vi "RSZVB Query Extension Unit Hardware Options.vi"(8 "error in (no error)":errorcluster {"code" format="%.0x"}, 11 "VISA session":refnum<visa-resource-name>) -> (0 "error out":errorcluster {"code" format="%.0x"}, 1 "Options":string, 3 "dup VISA session":refnum<visa-resource-name>)   [LabVIEW 2011]
doc: "Queries the hardware options of a connected extension unit ZVAXxx.\n\nRemote-control command(s):\nSYSTem:COMMunicate:RDEVice:EUNit:OPT?"
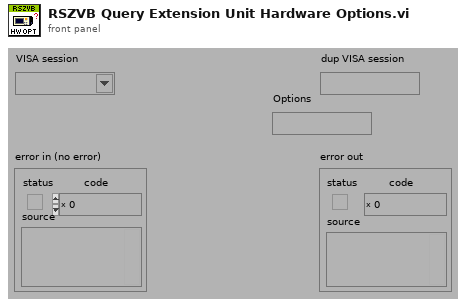
[diagram p1: front panel]
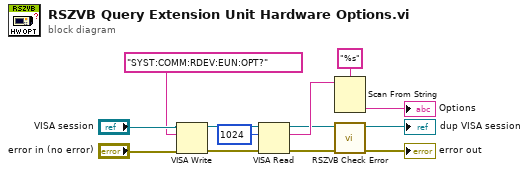
[diagram p0: block diagram]
diagram:
  n1 = VISA Write(VISA resource name="VISA session", write buffer="SYST:COMM:RDEV:EUN:OPT?", error in (no error)="error in (no error)") -> (VISA resource name out=w9:refnum<visa-resource-name>, error out=w10:errorcluster)  [unwired: 1 out]
  n2 = VISA Read(VISA resource name=w9, byte count=u32 1024, error in (no error)=w10) -> (VISA resource name out=w1:refnum<visa-resource-name>, read buffer=w6:string, error out=w4:errorcluster)  [unwired: 1 out]
  n3 = Scan From String(format string="%s", input string=w6) -> (output 1=→"Options":string)  [unwired: 3 in, 3 out]
  n4 = call "RSZVB Check Error.vi"("error in (no error)"=w4, "VISA session"=w1) -> ("error out"=→"error out":errorcluster, "dup VISA session"=→"dup VISA session":refnum<visa-resource-name>)  [unwired: 8 in]
